vi "Generate Simulated Data.vi"(7 "Type de mode":bool, 8 "error in (no error)":T2 caption="entrée d'erreur (pas d'erreur)", 9 "Péri":tag="Dev1", 10 "Longueur d'onde":dbl, 11 "Type de signal":T1) -> (0 "error out":T2 caption="sortie d'erreur", 2 "Données du graphe":waveform(dbl)[](array[waveform]))   [LabVIEW 2018, in "Acquisition.lvlib"]
doc: "Génère des exemples de waveforms en fonction du type de signal dans l'entrée Configuration du matériel."
uses:
  Acquisition.lvlib
  Signal Type.ctl
  <vilib>/Analysis/baseanly.llb/Mean (DBL).vi
  <vilib>/Analysis/NI_AALBase.lvlib
panel:
  out "Graphe déroulant":dynamicdata(graph)
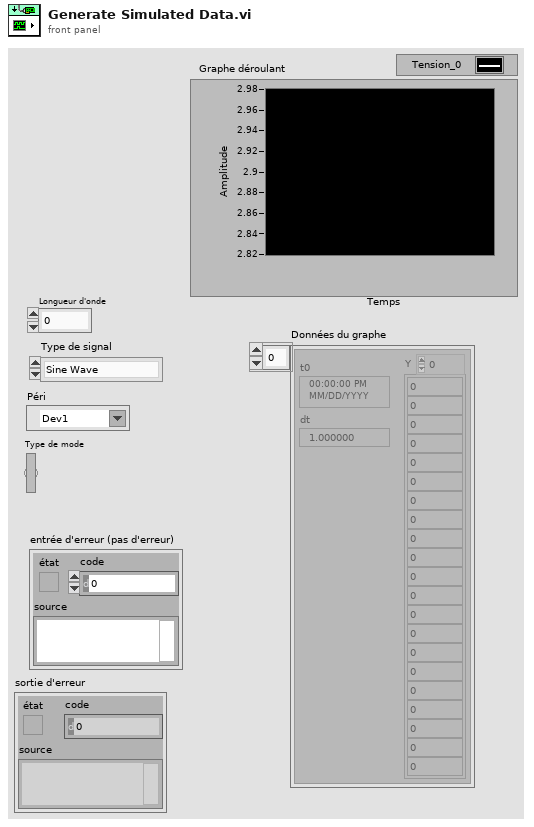
[diagram p1: front panel]
types:
  T1 = typedef "Acquisition.lvlib/Signal Type.ctl" = enum16{"Sine Wave", "Square with Noise", "Signal triangulaire", "Simulation DAQ"}
  T2 = cluster{"état":bool, "code":i32, "source":string}
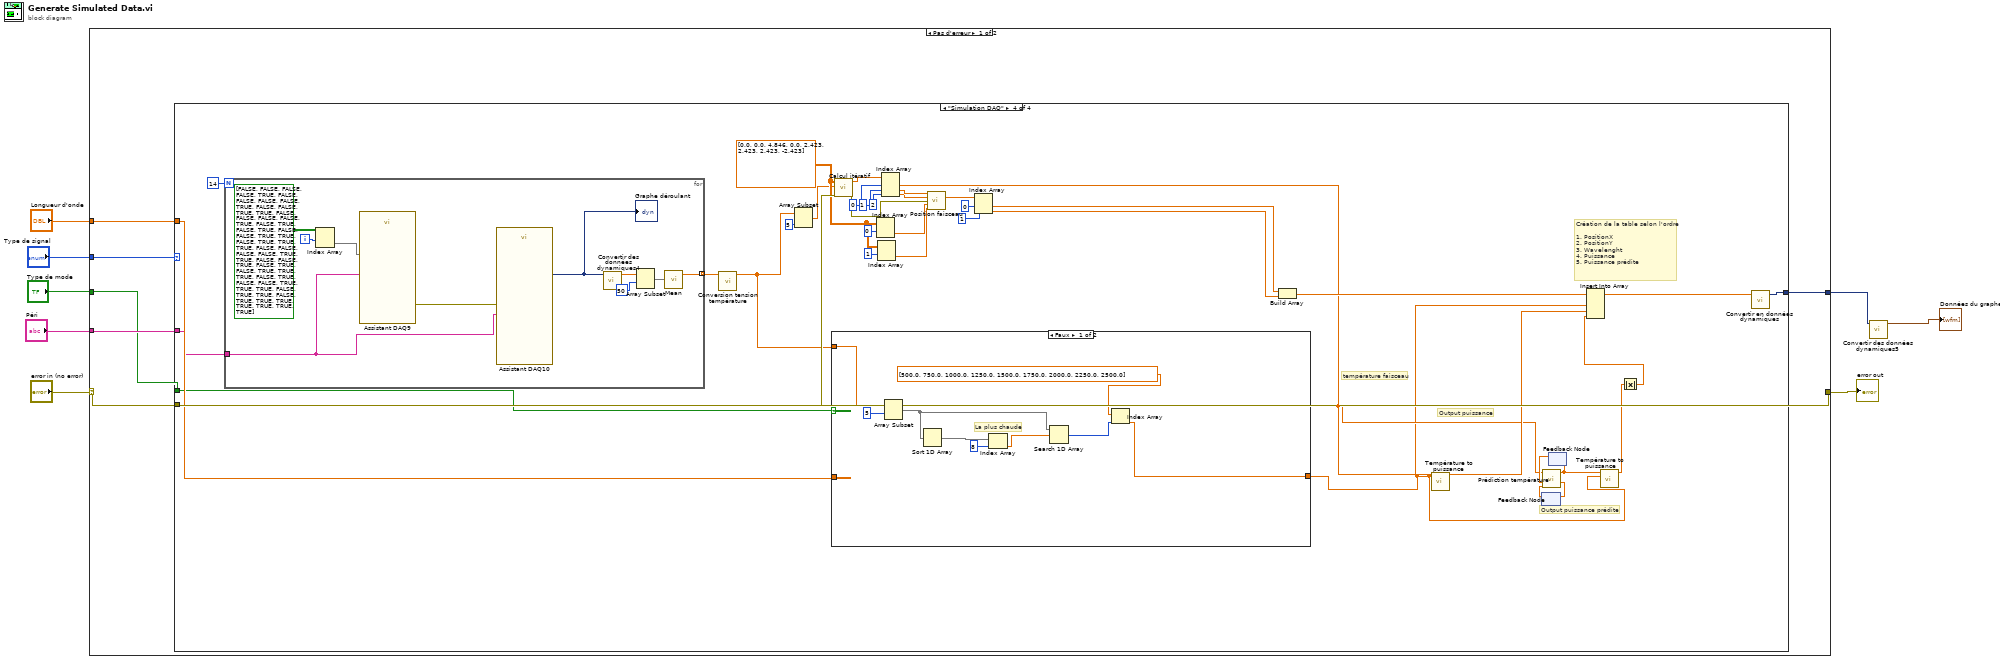
[diagram p0: block diagram]
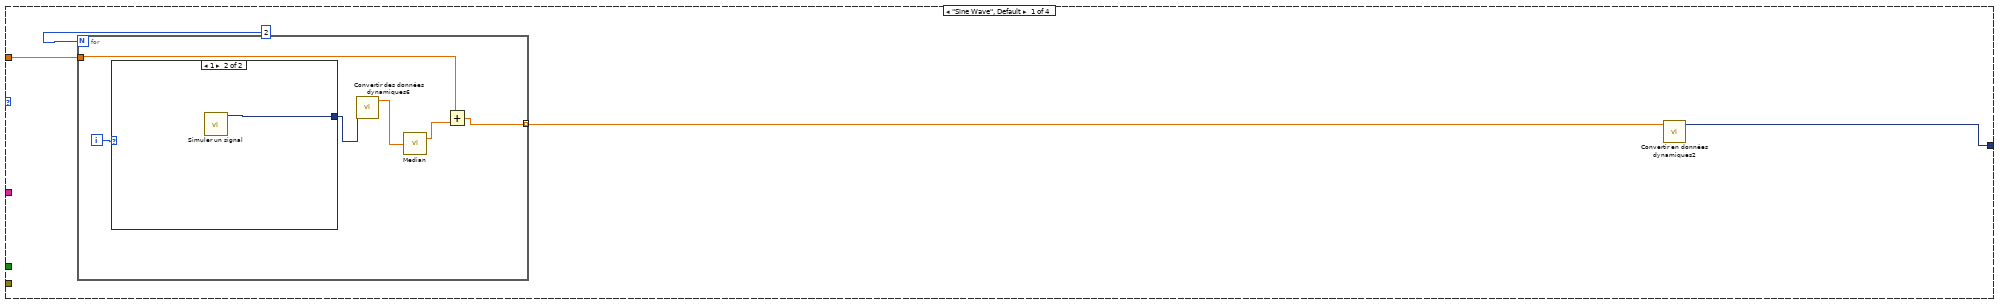
[diagram p2: hidden frame]
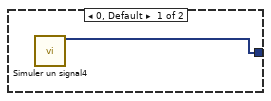
[diagram p3: hidden frame]
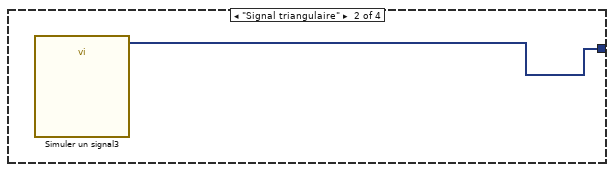
[diagram p4: hidden frame]
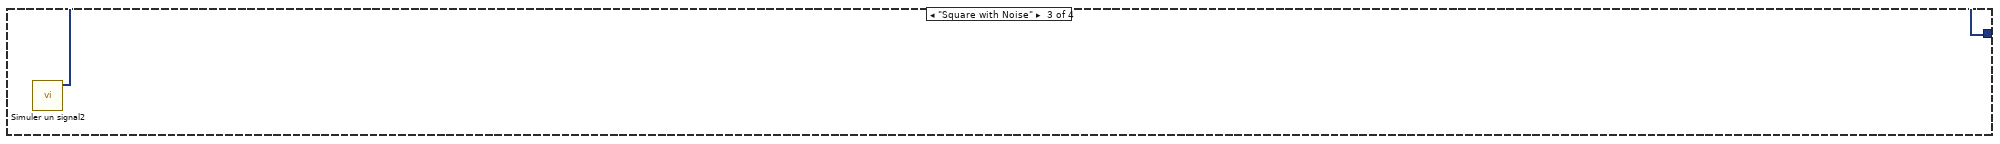
[diagram p5: hidden frame]
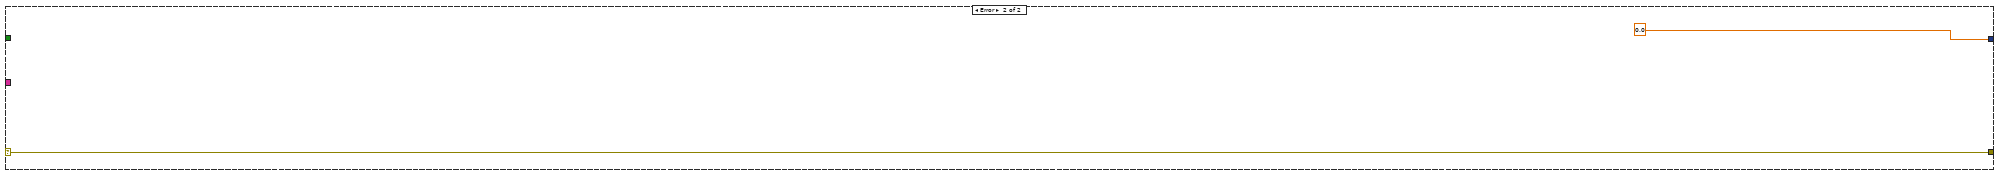
[diagram p7: hidden frame]
diagram:
  n1 = case shown="Pas d'erreur" "error in (no error)" {
    selector: "error in (no error)" -> [w9 w88]
    tunnel: [w9 w88] -> w7
    tunnel: "Type de signal" -> [w14 _]
    tunnel: [w13 0.0] -> w4
    tunnel: "Longueur d'onde" -> [w12 _]
    tunnel: "Péri" -> [w11 _]
    tunnel: "Type de mode" -> [w10 _]
    frame No Error {
      n2 = case shown="\"Simulation DAQ\"" w14 {
        tunnel: [w17 w27 w28 w65] -> w13
        tunnel: w12 -> [w16 _ _ w64]
        tunnel: w11 -> [_ _ _ w63]
        tunnel: w10 -> [_ _ _ w62]
        tunnel: w9 -> [_ _ _ w59]
        frame "Sine Wave", Default {
          n3 = for {
            N: 2 -> [_]
            tunnel: [w20] -> w15 mode=indexing
            tunnel: w16 -> [w19]
            i -> [w24]
            n4 = case shown="1" w24 {
              tunnel: [w25 w26] -> w23
              frame 0, Default {
                n5 = call "Simuler un signal4"() -> ("CC"=w25:dynamicdata)  [unwired: 14 in, 1 out]
              }
              frame 1 {
                n6 = call "Simuler un signal"() -> ("Sinus avec Bruit uniforme"=w26:dynamicdata)  [unwired: 14 in, 1 out]
              }
            }
            n7 = call "Convertir des données dynamiques6"("Dynamic Data Type"=w23) -> ("Array"=w22:dbl[])  [unwired: 3 in]
            n8 = call <vilib>:"Median.vi"("X"=w22) -> ("median"=w21:dbl)  [unwired: 1 out]
            n9 = Add(x=w19, y=w21) -> (x+y=w20:dbl)
          }
          n10 = call "Convertir en données dynamiques2"("Array"=w15) -> ("Dynamic Data Type"=w17:dynamicdata)  [unwired: 3 in]
        }
        frame "Signal triangulaire" {
          n11 = call "Simuler un signal3"() -> ("Triangle"=w27:dynamicdata)  [unwired: 14 in, 1 out]
        }
        frame "Square with Noise" {
          n12 = call "Simuler un signal2"() -> ("Square with Gaussian Noise"=w28:dynamicdata)  [unwired: 14 in, 1 out]
        }
        frame "Simulation DAQ" {
          w58 = dbl[][] [[0.0, 0.0], [4.846, 0.0], [2.423, 2.423], [2.423, -2.423]] ("Position des capteurs")
          # "température faisceau"
          # "Output puissance prédite"
          # "Création de la table selon l'ordre\n\n1. PositionX\n2. PositionY\n3. Wavelenght\n4. Puissance\n5. Puissance prédite"
          # "Output puissance"
          n13 = for {
            N: 14 -> [_]
            tunnel: [w78] -> w60 mode=indexing
            tunnel: w63 -> [w77]
            i -> [w84]
            n14 = Index Array(array=bool[][] [[FALSE, FALSE, FALSE, FALSE], [TRUE, FALSE, FALSE, FALSE], [FALSE, TRUE, FALSE, FALSE], [TRUE, TRUE, FALSE, FALSE], [FALSE, FALSE, TRUE, FALSE], [TRUE, FALSE, TRUE, FALSE], [FALSE, TRUE, TRUE, FALSE], [TRUE, TRUE, TRUE, FALSE], [FALSE, FALSE, FALSE, TRUE], [TRUE, FALSE, FALSE, TRUE], [FALSE, TRUE, FALSE, TRUE], [TRUE, TRUE, FALSE, TRUE], [FALSE, FALSE, TRUE, TRUE], [TRUE, FALSE, TRUE, TRUE], [FALSE, TRUE, TRUE, TRUE], [TRUE, TRUE, TRUE, TRUE]], index (row)=w84) -> (element=w83:bool[])  [unwired: 1 in]
            n15 = call "Assistant DAQ9"("data"=w83, "nom du périphérique"=w77) -> ("error out"=w86:errorcluster)  [unwired: 16 in, 1 out]
            n16 = call "Assistant DAQ10"("error in"=w86, "nom du périphérique"=w77) -> ("data"=w82:dynamicdata)  [unwired: 15 in, 2 out]
            "Graphe déroulant" <- w82
            n17 = call "Convertir des données dynamiques4"("Dynamic Data Type"=w82) -> ("Array"=w81:dbl[])  [unwired: 3 in]
            n18 = Array Subset(array=w81, index=50 ("indice")) -> (w79:dbl[])  [unwired: 1 in]
            n19 = call-poly <vilib>:"Mean.vi"("X"=w79) -> ("mean"=w78:dbl)  [unwired: 1 out]
          }
          n20 = call "Conversion tension température.vi"("Tension In"=w60) -> ("Température Out"=w29:dbl[])  [unwired: 10 in]
          n21 = Array Subset(array=w29, length=5 ("longueur")) -> (w33:dbl[])  [unwired: 1 in]
          n22 = case shown="Faux" w62 {
            tunnel: [w67 w76] -> w32
            tunnel: w64 -> [_ w76]
            tunnel: w29 -> [w75 _]
            frame False {
              # "La plus chaude"
              n23 = Array Subset(array=w75, index=5 ("indice")) -> (w70:dbl[])  [unwired: 1 in]
              n24 = Sort 1D Array(array=w70) -> (sorted array=w72:dbl[])
              n25 = Index Array(array=w72, index=8 ("indice")) -> (element=w71:dbl)
              n26 = Search 1D Array(1D array=w70, element=w71) -> (index of element=w69:i32)  [unwired: 1 in]
              n27 = Index Array(array=dbl[] [500.0, 750.0, 1000.0, 1250.0, 1500.0, 1750.0, 2000.0, 2250.0, 2500.0], index=w69) -> (element=w67:dbl)
            }
            frame True {
            }
          }
          n28 = call "Calcul itératif.vi"("error in (no error)"=w59, "Température capteur 1-2-3-4-Ambiant"=w33, "Position des capteurs"=w58) -> ("error out"=w40:T2, "DATA - T/R1/R2/R3"=w45:dbl[])  [unwired: 7 in]
          n29 = Index Array(array=w58, index (row)=0 ("indice (ligne)")) -> (element=w57:dbl[])  [unwired: 1 in]
          n30 = Index Array(array=w58, index (row)=1 ("indice (ligne)")) -> (element=w56:dbl[])  [unwired: 1 in]
          n31 = Index Array(array=w45, index #1=0, index #2=1 ("indice"), index #3=2 ("indice")) -> (element #1=w36:dbl, element #2=w44:dbl, element #3=w43:dbl)
          n32 = call "Position faisceau.vi"("R1"=w44, "R2"=w43, "error in (no error)"=w40, "Capteur 1"=w57, "Capteur 2"=w56) -> ("Coord"=w53:dbl[])  [unwired: 9 in, 1 out]
          n33 = Index Array(array=w53, index #1=0 ("indice"), index #2=1 ("indice")) -> (element #1=w50:dbl, element #2=w49:dbl)
          n34 = Build Array(w50, w49) -> (w42:dbl[])
          n35 = call "Température to puissance.vi"("Longueur d'onde"=w32, "Température max"=w36) -> ("Puissance"=w41:dbl)  [unwired: 9 in]
          n36 = feedback #1() -> (w39:dbl)  [unwired: 1 in]
          n37 = feedback #2() -> (w38:dbl)  [unwired: 1 in]
          n38 = call "Prédiction température.vi"("Temps -2"=w39, "Temps -1"=w38, "Temps 0"=w36) -> ("Temps-1"=w37:dbl, "Temps pred"=w35:dbl)  [unwired: 7 in]
          n39 = feedback-in #1(w37) -> ()
          n40 = feedback-in #2(w35) -> ()
          n41 = call "Température to puissance.vi"("Longueur d'onde"=w32, "Température max"=w35) -> ("Puissance"=w31:dbl)  [unwired: 9 in]
          n42 = Absolute Value(x=w31) -> (abs(x)=w30:dbl)
          n43 = Insert Into Array(array=w42, new element #1=w32, new element #2=w41, new element #3=w30) -> (w61:dbl[])  [unwired: 1 in]
          n44 = call "Convertir en données dynamiques"("Array"=w61) -> ("Dynamic Data Type"=w65:dynamicdata)  [unwired: 3 in]
        }
      }
    }
    frame Error {
    }
  }
  "error out" <- w7
  n45 = call "Convertir des données dynamiques5"("Dynamic Data Type"=w4) -> ("Array of Waveform"=→"Données du graphe":waveform(dbl)[])  [unwired: 3 in]
